vi "use_pick_line_or_format_stirng.vi"(11 "BD":string) -> (3 "Pick Line Node?":bool)   [LabVIEW 2018]
uses:
  <vilib>/regexp/Match Regular Expression.xnode
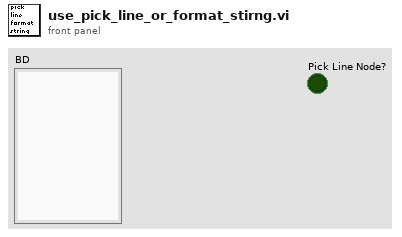
[diagram p1: front panel]
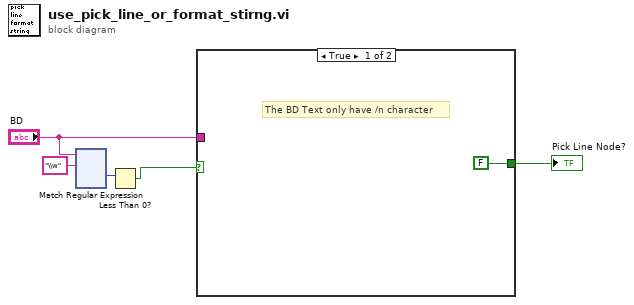
[diagram p0: block diagram]
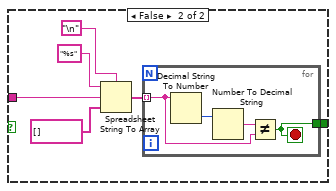
[diagram p2: hidden frame]
diagram:
  n1 = xnode "Match Regular Expression"("input string"="BD", "regular expression"="\\w") -> ("offset past match"=w2:i32)  [unwired: 2 in, 6 out]
  n2 = Less Than 0?(x=w2) -> (x < 0?=w1:bool)
  n3 = case shown="True" w1 {
    tunnel: [FALSE w8] -> w5
    tunnel: "BD" -> [_ w7]
    frame True {
      # "The BD Text only have /n character"
    }
    frame False {
      n4 = Spreadsheet String To Array(delimiter (Tab)="\n", format string="%s", spreadsheet string=w7, array type (2D Dbl)=string[] []) -> (array=w9:string[])
      n5 = for {
        tunnel: w9 -> [w14] mode=indexing
        tunnel: [w13] -> w8
        stop <- w13 stop-if-true
        n6 = Decimal String To Number(string=w14) -> (number=w16:i32)  [unwired: 3 out]
        n7 = Number To Decimal String(number=w16) -> (decimal integer string=w15:string)  [unwired: 1 out]
        n8 = Not Equal?(x=w15, y=w14) -> (x != y?=w13:bool)
      }
    }
  }
  "Pick Line Node?" <- w5
